vi "Request Data JSON.vi"(8 "error in (no error)":errorcluster, 11 "SetSceneItemEnabled in":refnum<class "SetSceneItemEnabled.lvclass">) -> (0 "error out":errorcluster, 2 "Request Data JSON":string, 3 "SetSceneItemEnabled out":refnum<class "SetSceneItemEnabled.lvclass">)   [LabVIEW 2020, in "obs-websocket.lvlib" / "SetSceneItemEnabled.lvclass"]
uses:
  SetSceneItemEnabled.lvclass
  SetSceneItemEnabled.lvclass/SetSceneItemEnabled.ctl
  51bafc63-6a1d-461f-bad9-5a896d7765c8.vi
  <vilib>/JDP Science/JSONtext/Variant to JSON Text.vi
  <vilib>/JDP Science/JSONtext/LVClass Serializer/JSONtext LVClass Serializer.lvclass
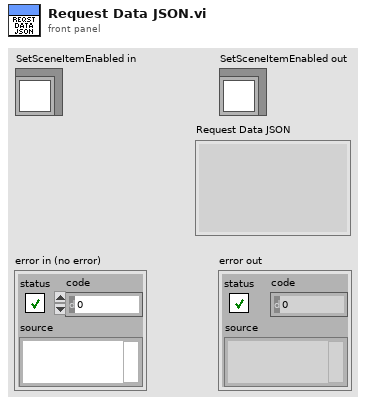
[diagram p1: front panel]
types:
  T1 = cluster{"sceneName":string, "sceneItemId":i32, "sceneItemEnabled":bool}
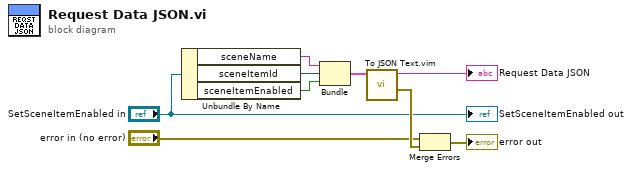
[diagram p0: block diagram]
diagram:
  n1 = Unbundle By Name("SetSceneItemEnabled in") -> ("sceneName"=w7:string, "sceneItemId"=w6:i32, "sceneItemEnabled"=w5:bool)
  n2 = Bundle("sceneName"=w7, "sceneItemId"=w6, "sceneItemEnabled"=w5) -> (w4:T1)  [unwired: 1 in]
  n3 = call "To JSON Text.vim"("Anything"=w4) -> ("error out"=w9:errorcluster, "<JSON>"=→"Request Data JSON":string)  [unwired: 9 in]
  n4 = Merge Errors("error in (no error)", w9) -> (→"error out":errorcluster)
  "SetSceneItemEnabled out" <- "SetSceneItemEnabled in"
